vi "Rename Library.vi"(6 "Rename Library File Path":path, 8 "error in":errorcluster, 9 "Name Library File Path":path, 10 "Project:Active Project":refnum<vi>) -> (0 "error out":errorcluster)   [LabVIEW 2021, in "_Rename.lvlib" / "_Rename.lvclass"]
uses:
  _Rename.lvclass
  _Rename.lvclass/_Rename.ctl
  <vilib>/Utility/EditLVLibs/Edit LVLibs.lvlib
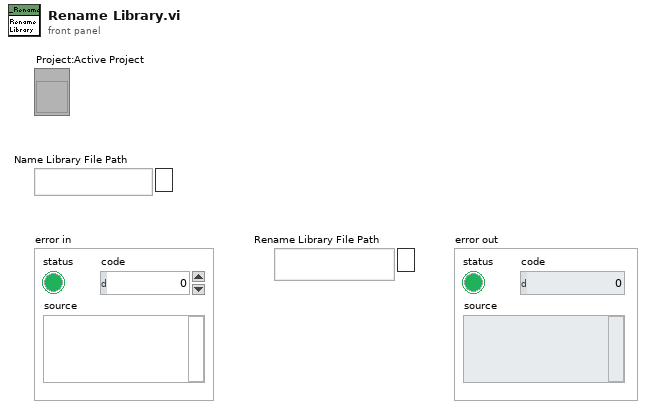
[diagram p1: front panel]
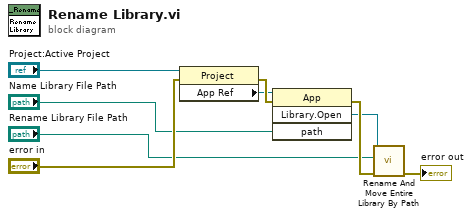
[diagram p0: block diagram]
diagram:
  n1 = property class="Project"(reference="Project:Active Project", error in="error in") -> (error out=w7:errorcluster, "App Ref"=w6:refnum<vi>)  [unwired: 1 out]
  n2 = invoke class="App" method="Library.Open"(reference=w6, error in=w7, "path"="Name Library File Path") -> (error out=w8:errorcluster, "Open Library"=w5:refnum<vi>)  [unwired: 1 in, 2 out]
  n3 = call <vilib>:"Rename And Move Entire Library By Path.vi"("error in (no error)"=w8, "New library path"="Rename Library File Path", "Library ref in"=w5) -> ("error out"=→"error out":errorcluster)  [unwired: 7 in, 1 out]
